vi "Manual Time Stamp Calculation Example.vi"() -> ()   [LabVIEW 2019]
panel:
  out "Time Stamp\n(Not based on System Clock)":timestamp
  out "Loop Count":dbl
  in  "stop":bool
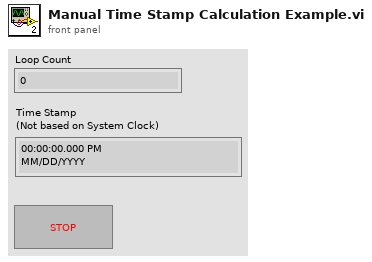
[diagram p1: front panel]
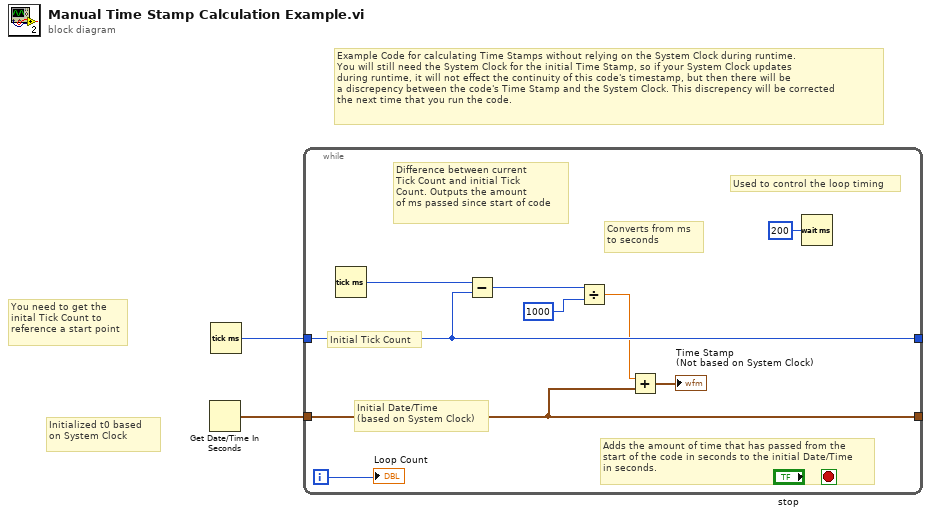
[diagram p0: block diagram]
diagram:
  # "Example Code for calculating Time Stamps without relying on the System Clock during runtime. \nYou will still need the System Clock for the initial Time Stamp, so if your System Clock updates\nduring runtime, it will not effect the continuity of this code's timestamp, but then there will be \na discrepency between the code's Time Stamp and the System Clock. This discrepency will be corrected\nthe next time that you run the code."
  # "You need to get the \ninital Tick Count to \nreference a start point"
  # "Initialized t0 based\non System Clock"
  n1 = Get Date/Time In Seconds() -> (seconds since 1Jan1904=w1:timestamp)
  n2 = Tick Count (ms)() -> (millisecond timer value=w2:u32)
  n3 = while {
    tunnel: w2 -> [w9]
    tunnel: [w9] -> _
    tunnel: [w8] -> _
    tunnel: w1 -> [w8]
    i -> [w3]
    stop <- "stop" stop-if-true
    # "Adds the amount of time that has passed from the\nstart of the code in seconds to the initial Date/Time\nin seconds."
    # "Initial Date/Time\n(based on System Clock)"
    # "Converts from ms\nto seconds"
    # "Difference between current \nTick Count and initial Tick\nCount. Outputs the amount\nof ms passed since start of code"
    # "Initial Tick Count"
    # "Used to control the loop timing"
    n4 = Tick Count (ms)() -> (millisecond timer value=w10:u32)
    n5 = Subtract(x=w10, y=w9) -> (x-y=w6:u32)
    n6 = Divide(x=w6, y=u32 1000) -> (x/y=w4:dbl)
    n7 = Add(x=w4, y=w8) -> (x+y=→"Time Stamp\n(Not based on System Clock)":timestamp)
    n8 = Wait (ms)(milliseconds to wait=u32 200) -> ()  [unwired: 1 out]
    "Loop Count" <- w3
  }
